vi "filter.teams.and.chars.per.volume.vi"() -> ()   [LabVIEW 2024]
uses:
  definitions/comicvine_issue.generic_credit.ctl
panel:
  in  "Threshold":dbl
  out "Chars Ranked":cluster{"size":i32, "character_credit":T1}[](array[cluster])
  out "Teams Ranked":cluster{"size":i32, "character_credit":T1}[](array[cluster])
  out "count_of_issues":i32
  out "error out":errorcluster
  in  "error in":errorcluster
  in  "volume json":path
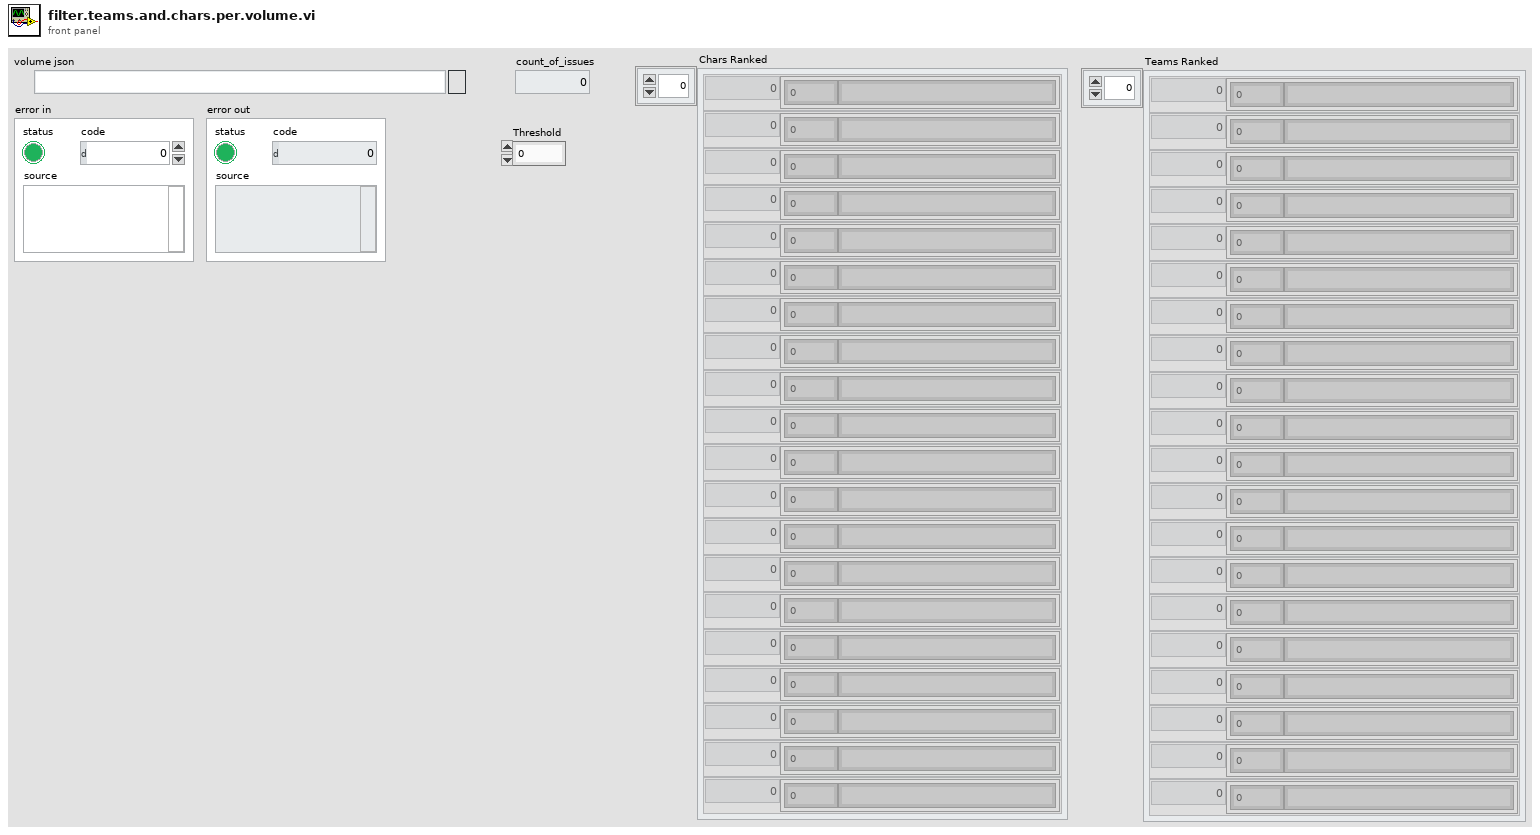
[diagram p1: front panel]
types:
  T1 = typedef "comicvine_issue.generic_credit.ctl" = cluster{"id":i32, "name":string}
  T2 = typedef "local_volume.ctl" = cluster{"id":i32, "name":string, "sortable_name":string, "aliases":string[], "description":string, "site_detail_url":string, "count_of_issues":i32, "start_year":i32, "publisher_id":i32, "issue_ids":i32[], "date_last_updated":timestamp, "volume":i32, "cv_id":string}
  T3 = typedef "local_issue.ctl" = cluster{"cover_date":timestamp, "id":i32, "cv_id":string, "name":string, "sortable_name":string, "issue_number":string, "deck":string, "description":string, "volume":T1, "store_date":timestamp, "date_last_updated":timestamp, "site_detail_url":string, "cover_url":string, "associated_images":T4[], "characters":T1[], "concepts":T1[], "creators":T5[], "storyArcs":T1[], "teams":T1[]}
  T4 = typedef "comicvine_issue.associated_image.ctl" = cluster{"original_url":string, "id":i32}
  T5 = typedef "comicvine_issue.person_credit.ctl" = cluster{"id":i32, "name":string, "role":string}
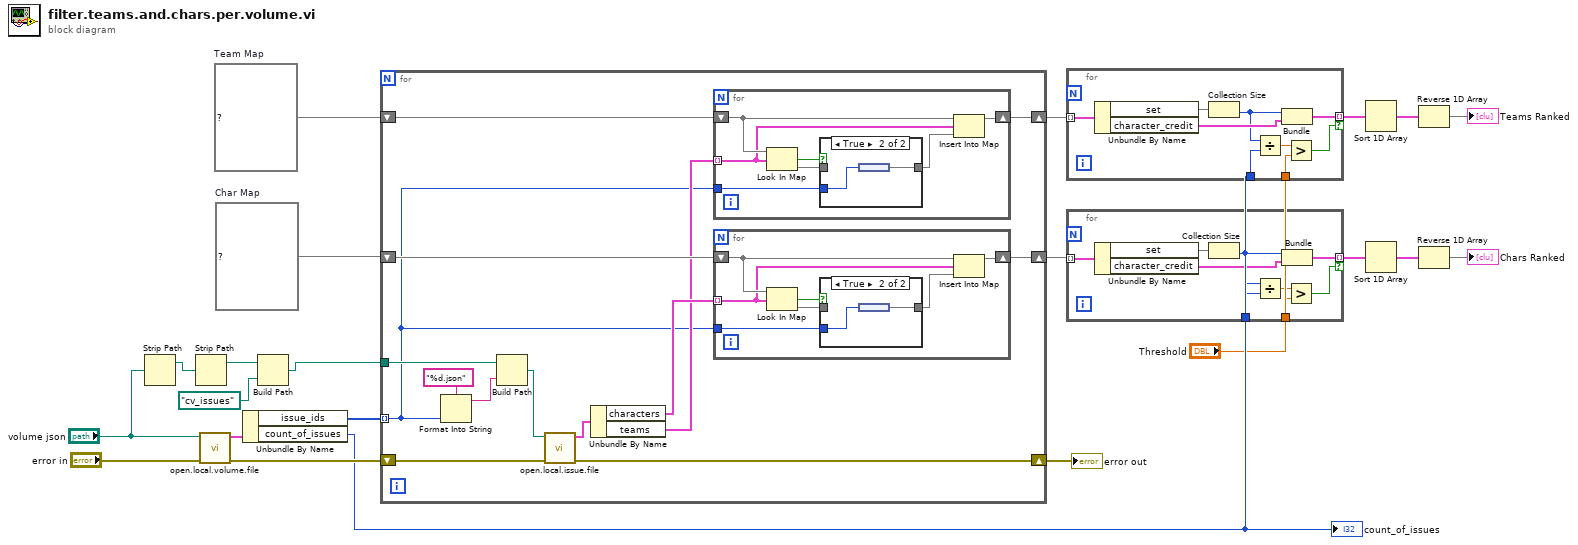
[diagram p0: block diagram]
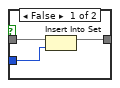
[diagram p2: hidden frame]
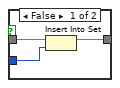
[diagram p3: hidden frame]
diagram:
  w11 = map{T1, set{i32}} {}  # Team Map
  w12 = map{T1, set{i32}} {}  # Char Map
  n1 = Strip Path(path="volume json") -> (stripped path=w19:path)  [unwired: 1 out]
  n2 = Strip Path(path=w19) -> (stripped path=w18:path)  [unwired: 1 out]
  n3 = call "open.local.volume.file.vi"("error in (no error)"="error in", "volume json"="volume json") -> ("error out"=w14:errorcluster, "volume"=w22:T2)  [unwired: 8 in]
  n4 = Unbundle By Name(w22) -> ("issue_ids"=w16:i32[], "count_of_issues"=w2:i32)
  "count_of_issues" <- w2
  n5 = Build Path(base path=w18, name or relative path=path "cv_issues") -> (appended path=w15:path)
  n6 = for {
    tunnel: w16 -> [w24] mode=indexing
    tunnel: w15 -> [w35]
    shift-right: [w31] -> w13
    shift-left: w14 -> [w32]
    shift-right: [w27] -> w4
    shift-left: w12 -> [w29]
    shift-right: [w23] -> w10
    shift-left: w11 -> [w26]
    n7 = Format Into String(format string="%d.json", w24) -> (resulting string=w34:string)  [unwired: 2 in, 1 out]
    n8 = Build Path(base path=w35, name or relative path=w34) -> (appended path=w33:path)
    n9 = call "open.local.issue.file.vi"("error in (no error)"=w32, "volume json"=w33) -> ("error out"=w31:errorcluster, "issue"=w30:T3)  [unwired: 8 in]
    n10 = Unbundle By Name(w30) -> ("characters"=w28:T1[], "teams"=w25:T1[])
    n11 = for {
      shift-right: [w39] -> w23
      shift-left: w26 -> [w40]
      tunnel: w25 -> [w38] mode=indexing
      tunnel: w24 -> [w41]
      n12 = Look In Map(map=w40, key=w38) -> (key not found?=w43:bool, value=w42:set{i32})  [unwired: 1 in]
      n13 = case shown="True" w43 {
        tunnel: w42 -> [w46 _]
        tunnel: w41 -> [w45 w48]
        tunnel: [w44 w47] -> w37
        frame False {
          n14 = Insert Into Set(10:w45, 11:w46) -> (3:w44:set{i32})  [unwired: 1 out]
        }
        frame True {
          n15 = node(w48) -> (w47:set{i32})
        }
      }
      n16 = Insert Into Map(map in=w40, key=w38, value=w37) -> (map out=w39:map{T1, set{i32}})  [unwired: 2 out]
    }
    n17 = for {
      shift-right: [w51] -> w27
      shift-left: w29 -> [w52]
      tunnel: w28 -> [w50] mode=indexing
      tunnel: w24 -> [w53]
      n18 = Look In Map(map=w52, key=w50) -> (key not found?=w55:bool, value=w54:set{i32})  [unwired: 1 in]
      n19 = case shown="True" w55 {
        tunnel: w54 -> [w58 _]
        tunnel: w53 -> [w57 w60]
        tunnel: [w56 w59] -> w49
        frame False {
          n20 = Insert Into Set(10:w57, 11:w58) -> (3:w56:set{i32})  [unwired: 1 out]
        }
        frame True {
          n21 = node(w60) -> (w59:set{i32})
        }
      }
      n22 = Insert Into Map(map in=w52, key=w50, value=w49) -> (map out=w51:map{T1, set{i32}})  [unwired: 2 out]
    }
  }
  "error out" <- w13
  n23 = for {
    tunnel: w10 -> [w69] mode=indexing
    tunnel: [w66] -> w9 mode=indexing if=w61
    tunnel: w2 -> [w64]
    tunnel: "Threshold" -> [w62]
    n24 = Unbundle By Name(w69) -> ("set"=w68:set{i32}, "character_credit"=w67:T1)
    n25 = Collection Size(1:w68) -> (0:w63:i32)
    n26 = Divide(x=w63, y=w64) -> (x/y=w65:dbl)
    n27 = Bundle("size"=w63, "character_credit"=w67) -> (w66:cluster{"size":i32, "character_credit":T1})  [unwired: 1 in]
    n28 = Greater?(x=w65, y=w62) -> (0:w61:bool)
  }
  n29 = for {
    tunnel: w4 -> [w78] mode=indexing
    tunnel: [w75] -> w3 mode=indexing if=w70
    tunnel: w2 -> [w73]
    tunnel: "Threshold" -> [w71]
    n30 = Unbundle By Name(w78) -> ("set"=w77:set{i32}, "character_credit"=w76:T1)
    n31 = Collection Size(1:w77) -> (0:w74:i32)
    n32 = Divide(x=w74, y=w73) -> (x/y=w72:dbl)
    n33 = Bundle("size"=w74, "character_credit"=w76) -> (w75:cluster{"size":i32, "character_credit":T1})  [unwired: 1 in]
    n34 = Greater?(x=w72, y=w71) -> (0:w70:bool)
  }
  n35 = Sort 1D Array(array=w9) -> (sorted array=w8:cluster{"size":i32, "character_credit":T1}[])
  n36 = Sort 1D Array(array=w3) -> (sorted array=w5:cluster{"size":i32, "character_credit":T1}[])
  n37 = Reverse 1D Array(array=w8) -> (reversed array=→"Teams Ranked":cluster{"size":i32, "character_credit":T1}[])
  n38 = Reverse 1D Array(array=w5) -> (reversed array=→"Chars Ranked":cluster{"size":i32, "character_credit":T1}[])
